vi "Wait on Connection State.vi"(8 "error in (no error)":errorcluster, 9 "Timeout ms (-1)":i32=-1, 10 "Connection State":T1, 11 "TCP Client in":refnum<class "TCP Client.lvclass">) -> (0 "error out":errorcluster, 1 "Timed Out?":bool, 3 "TCP Client out":refnum<class "TCP Client.lvclass">)   [LabVIEW 2020, in "Stream-TCP.lvlib" / "TCP Client.lvclass"]
uses:
  TCP Client.lvclass
  Connection State.ctl
  lv-trace/Trace/Trace.lvlib
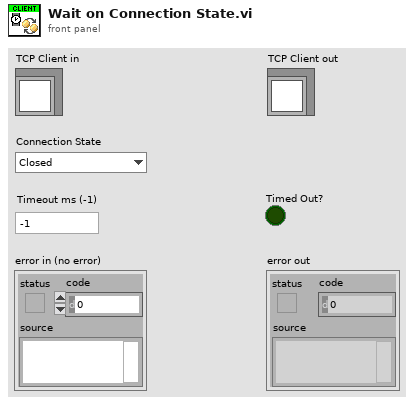
[diagram p1: front panel]
types:
  T1 = typedef "Stream-TCP.lvlib/TCP Client.lvclass/Connection State.ctl" = enum16{"Closed", "Idle", "Connecting", "Connected", "Shutdown"}
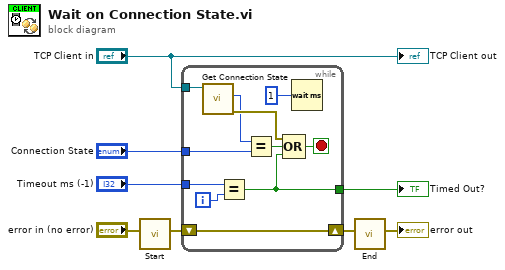
[diagram p0: block diagram]
diagram:
  n1 = call "Start.vi"("error in (no error)"="error in (no error)") -> ("error out"=w3:errorcluster)  [unwired: 10 in]
  n2 = while {
    tunnel: "Connection State" -> [w17]
    tunnel: "TCP Client in" -> [w18]
    tunnel: "Timeout ms (-1)" -> [w11]
    tunnel: [w10] -> w5
    shift-right: [w9] -> w2
    shift-left: w3 -> [w9]
    i -> [w12]
    stop <- w14 stop-if-true
    n3 = call "Get Connection State.vi"("TCP Client in"=w18) -> ("error out"=w19:errorcluster, "State"=w16:T1)  [unwired: 8 in, 1 out]
    n4 = Equal?(x=w11, y=w12) -> (x = y?=w10:bool)
    n5 = Equal?(x=w16, y=w17) -> (x = y?=w15:bool)
    n6 = Compound Arithmetic op=OR(w19, w15, w10) -> (w14:bool)
    n7 = Wait (ms)(milliseconds to wait=u32 1) -> ()  [unwired: 1 out]
  }
  "Timed Out?" <- w5
  n8 = call "End.vi"("error in (no error)"=w2) -> ("error out"=→"error out":errorcluster)  [unwired: 10 in]
  "TCP Client out" <- "TCP Client in"
